vi "Find No Graves with Empty VI.vi"(8 "Error In":errorcluster) -> (0 "Error Out":errorcluster)   [LabVIEW 2018, in "Tests.lvlib" / "Toolkit.lvlib" / "Integration.lvlib"]
uses:
  Integration.lvlib
  <vilib>/addons/_JKI Toolkits/Caraya/classes/Test/Test.lvclass
  <vilib>/addons/_JKI Toolkits/Caraya/classes/Assert/Assert.lvclass
  src/Toolkit/Toolkit.lvlib
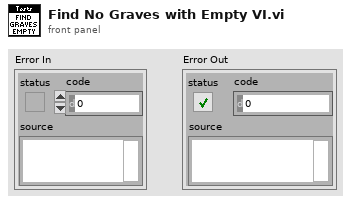
[diagram p1: front panel]
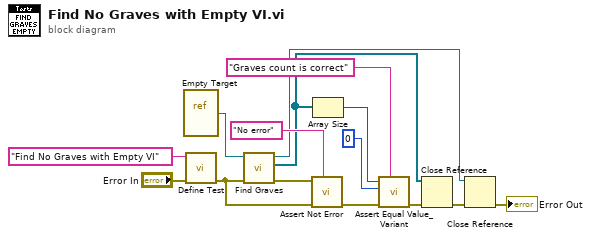
[diagram p0: block diagram]
diagram:
  n1 = vi-ref "Empty Target.vi"() -> (w1:refnum<vi>)
  n2 = call <vilib>:"Define Test.vi"("error in (no error)"="Error In", "Label (VI Title)"="Find No Graves with Empty VI") -> ("error out"=w6:errorcluster)  [unwired: 9 in]
  n3 = call "Find Graves.vi"("Error In"=w6, "VI In"=w1) -> ("Error Out"=w15:errorcluster, "Graves"=w4:refnum<vi>[], "VI Out"=w7:refnum<vi>)  [unwired: 7 in]
  n4 = call <vilib>:"Assert Not Error.vi"("Label"="No error", "error in (no error)"=w6, "Not Error?"=w15) -> ("error out"=w12:errorcluster)  [unwired: 8 in]
  n5 = Array Size(array=w4) -> (size(s)=w3:i32)
  n6 = call <vilib>:"Assert Equal Value_Variant.vi"("Label"="Graves count is correct", "error in (no error)"=w12, "Y"=0 ("size(s)"), "X"=w3) -> ("error out"=w9:errorcluster)  [unwired: 7 in]
  n7 = Close Reference(reference=w4, error in (no error)=w9) -> (error out=w5:errorcluster)
  n8 = Close Reference(reference=w7, error in (no error)=w5) -> (error out=→"Error Out":errorcluster)
